vi "Test GUI Loader.vi"() -> ()   [LabVIEW 2014]
uses:
  General/Controls/GUI Types.ctl
panel:
  in  "Quit":bool
  in  "OK Button":bool
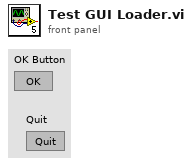
[diagram p1: front panel]
types:
  T1 = typedef "GUI Types.ctl" = enum16{"Mosaic GUI", "Vibratome GUI"}
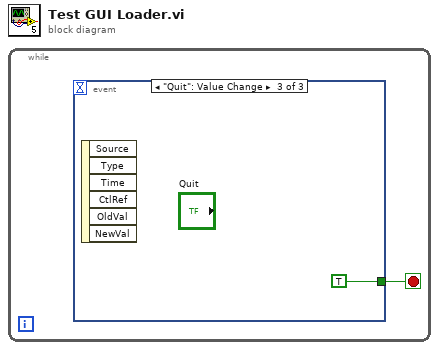
[diagram p0: block diagram]
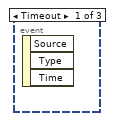
[diagram p2: hidden frame]
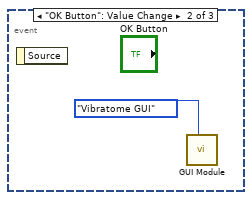
[diagram p3: hidden frame]
diagram:
  n1 = while {
    stop <- w1 stop-if-true
    n2 = event shown="[2] \"Quit\": Value Change" {
      selector: _ -> [_ _ _]
      dyn-events: _ -> [_ _ _]
      timeout: _ -> [_ _ _]
      tunnel: [_ _ TRUE] -> w1
      event Timeout {
        n3 = event-data() -> ()  [unwired: 1 in, 3 out]
      }
      event "OK Button": Value Change {
        n4 = event-data() -> ()  [unwired: 1 in, 1 out]
        n5 = call "GUI Module.vi"(7:GUI_Types."Vibratome GUI") -> ()  [unwired: 10 in, 1 out]
      }
      event "Quit": Value Change {
        n6 = event-data() -> ()  [unwired: 1 in, 6 out]
      }
    }
  }
